vi "grouping.vi"() -> ()   [LabVIEW 2023]
panel:
  in  "O2":cluster{"y2":dbl}
  in  "O1":cluster{"y1":dbl}
  in  "x2":dbl
  in  "x1":dbl
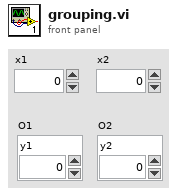
[diagram p1: front panel]
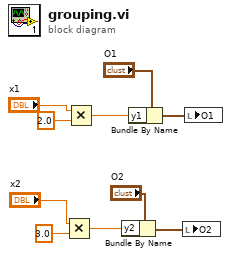
[diagram p0: block diagram]
diagram:
  n1 = Multiply(x="x2", y=3.0) -> (x*y=w2:dbl)
  n2 = Multiply(x="x1", y=2.0) -> (x*y=w6:dbl)
  n3 = Bundle By Name(cluster="O2", "y2"=w2) -> (w1:cluster{"y2":dbl})
  n4 = Bundle By Name(cluster="O1", "y1"=w6) -> (w9:cluster{"y1":dbl})
  n5 = local write "O2"(w1) -> ()
  n6 = local write "O1"(w9) -> ()
